vi "CliGetPduLength.vi"(0 "ref in":u64, 11 "error in (no error)":errorcluster) -> (4 "ref out":u64, 6 "Result":i32, 13 "Negotiated":i32, 14 "Requested":i32, 15 "error out":errorcluster)   [LabVIEW 2020, in "Snap7.lvlib"]
uses:
  Snap7.lvlib
  windows/lv_snap7.dll
panel:
  in  "var Negotiated":i32
  in  "var requested":i32
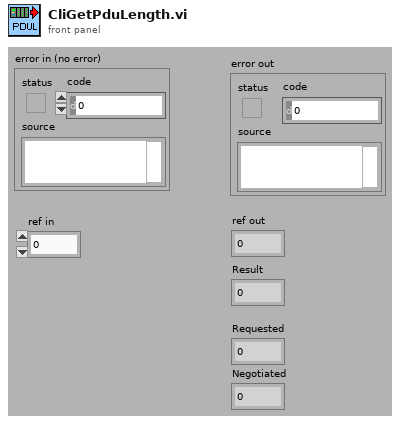
[diagram p1: front panel]
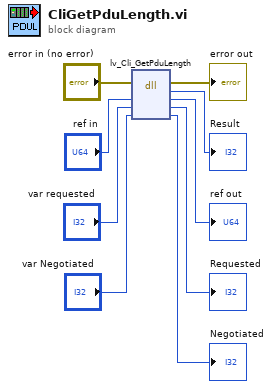
[diagram p0: block diagram]
diagram:
  n1 = dll-call lib="PTH2iabs CUsersFeng项目HLCEPS300-1老性能试验台SourcesSnap7libwindowslv_snap7.dll" fn="lv_Cli_GetPduLength"(error in="error in (no error)", "Client"="ref in", "Requested"="var requested", "Negotiated"="var Negotiated") -> (error out=→"error out":errorcluster, "return type"=→"Result":i32, "Client"=→"ref out":u64, "Requested"=→"Requested":i32, "Negotiated"=→"Negotiated":i32)  [unwired: 2 in, 1 out]
